vi "Video Displays.vi"() -> ()   [LabVIEW 2017]
uses:
  VideoWindowsCommand.ctl
panel:
  in  "Video Feed 2":enum16{"Camera 1", "Camera2", "Mobile"}(ring)=enum."Camera2"
  in  "MozillaBrowser 2":refnum<k7>(container)
  in  "Video Feed":enum16{"Camera 1", "Camera2", "Mobile"}(ring)
  in  "MozillaBrowser":refnum<k7>(container)
  in  "Exit":bool
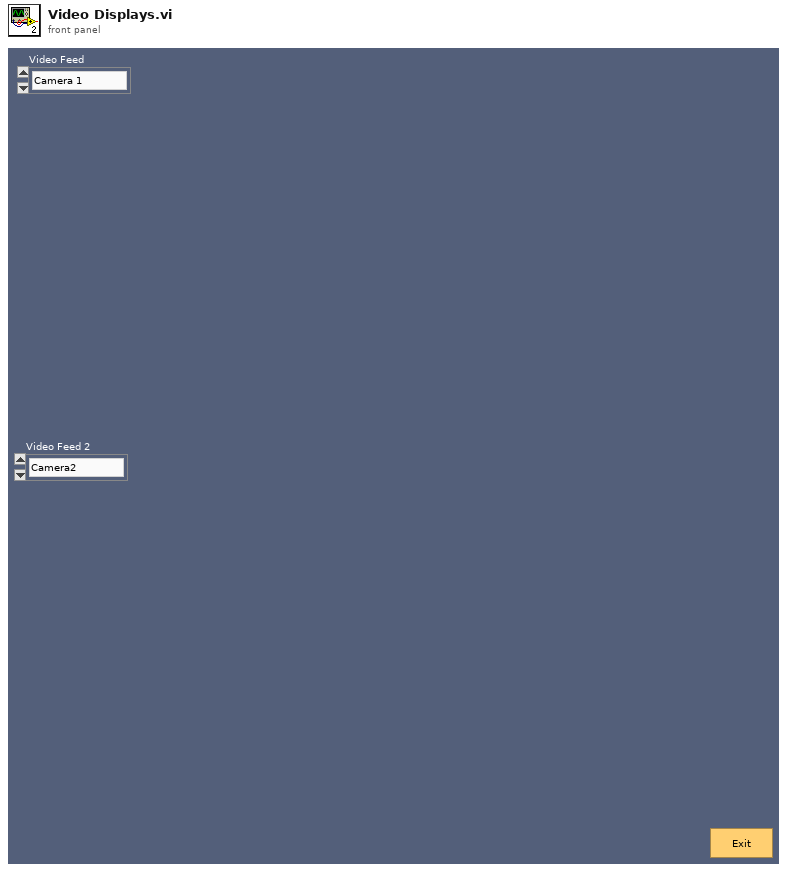
[diagram p1: front panel]
types:
  T1 = typedef "VideoWindowsCommand.ctl" = cluster{"Position":cluster{"Right":i32, "Bottom":i32}, "Exit":bool, "MoveToFront":bool}
  T2 = typedef "LVRectTypeDef.ctl" = cluster{"Left":i16, "Top":i16, "Right":i16, "Bottom":i16}
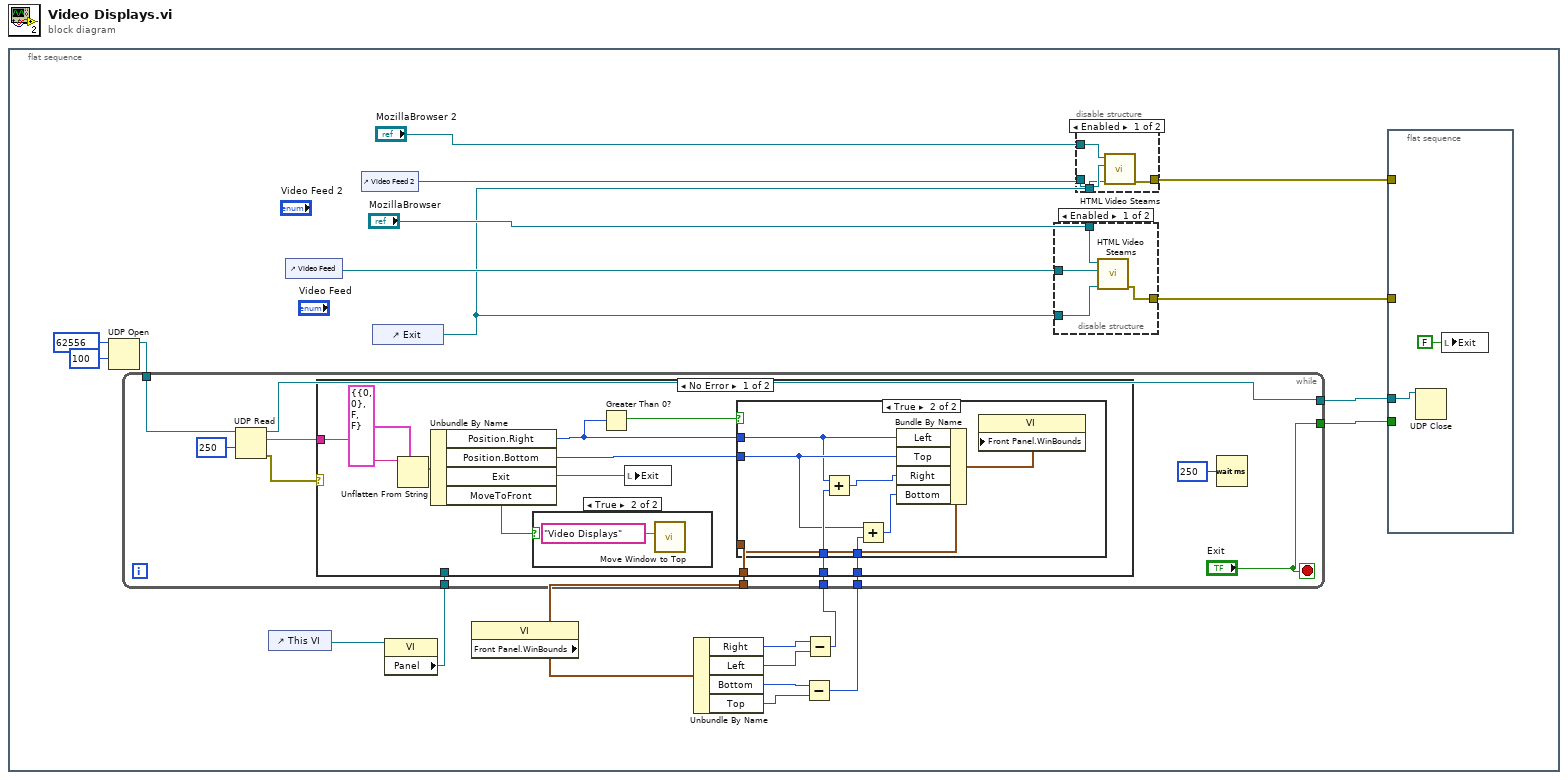
[diagram p0: block diagram]
diagram:
  n1 = flat-sequence {
    frame #0 {
      n2 = UDP Open(9:100 ("timeout ms (25000)"), 11:u16 62556 ("port")) -> (port=w12:refnum<k16>)  [unwired: 3 in, 2 out]
      n3 = control-ref of="This VI"() -> (w11:refnum<vi>)
      n4 = control-ref of="Video Feed"() -> (w20:refnum<vi>)
      n5 = control-ref of="Video Feed 2"() -> (w18:refnum<vi>)
      n6 = control-ref of="Exit"() -> (w14:refnum<vi>)
      n7 = property class="VI"(reference=w11) -> ("Panel"=w10:refnum<vi>)  [unwired: 1 in, 2 out]
      n8 = property class="VI"() -> ("Front Panel.WinBounds"=w3:T2)  [unwired: 2 in, 2 out]
      n9 = Unbundle By Name(w3) -> ("Right"=w6:i16, "Left"=w7:i16, "Bottom"=w4:i16, "Top"=w5:i16)
      n10 = Subtract(x=w4, y=w5) -> (x-y=w1:i16)
      n11 = Subtract(x=w6, y=w7) -> (x-y=w2:i16)
      n12 = while {
        tunnel: ["Exit"] -> w15
        tunnel: w12 -> [w32]
        tunnel: w10 -> [w28]
        tunnel: [w27] -> w9
        tunnel: w3 -> [w26]
        tunnel: w2 -> [w25]
        tunnel: w1 -> [w24]
        stop <- "Exit" stop-if-true
        n13 = UDP Read(connection ID=w32, timeout ms (25000)=250) -> (data out=w29:string, error out=w30:errorcluster, 3:w27:refnum<k16>)  [unwired: 2 in, 2 out]
        n14 = case shown="No Error" w30 {
          tunnel: w29 -> [w45 _]
          tunnel: w28 -> [_ _]
          tunnel: w26 -> [w41 _]
          tunnel: w25 -> [w40 _]
          tunnel: w24 -> [w38 _]
          frame No Error {
            n15 = Unflatten From String(type=T1 {"Position"={"Right"=0, "Bottom"=0}, "Exit"=FALSE, "MoveToFront"=FALSE}, binary string=w45) -> (value=w43:T1)  [unwired: 3 in, 2 out]
            n16 = Unbundle By Name(w43) -> ("Position.Right"=w37:i32, "Position.Bottom"=w39:i32, "Exit"=w42:bool, "MoveToFront"=w35:bool)
            n17 = case shown="True" w35 {
              frame False {
              }
              frame True {
                n18 = call "Move Window to Top.vi"("window name (\"\")"="Video Displays" ("window name (\"\")")) -> ()  [unwired: 5 in, 2 out]
              }
            }
            n19 = Greater Than 0?(x=w37) -> (x > 0?=w36:bool)
            n20 = local write "Exit"(w42) -> ()
            n21 = case shown="True" w36 {
              tunnel: w41 -> [_ w54]
              tunnel: w40 -> [_ w53]
              tunnel: w39 -> [_ w51]
              tunnel: w38 -> [_ w50]
              tunnel: w37 -> [_ w47]
              frame False {
              }
              frame True {
                n22 = Add(x=w47, y=w53) -> (x+y=w52:i32)
                n23 = Add(x=w51, y=w50) -> (x+y=w49:i32)
                n24 = Bundle By Name(cluster=w54, "Left"=w47, "Top"=w51, "Right"=w52, "Bottom"=w49) -> (w48:T2)
                n25 = property class="VI"("Front Panel.WinBounds"=w48) -> ()  [unwired: 2 in, 2 out]
              }
            }
          }
          frame Error {
          }
        }
        n26 = Wait (ms)(milliseconds to wait=u32 250) -> ()  [unwired: 1 out]
      }
      n27 = disable-structure shown="Enabled" {
        disable-tunnel: "MozillaBrowser" -> [w58 _]
        disable-tunnel: [w57 _] -> w16
        disable-tunnel: w20 -> [w56 _]
        disable-tunnel: w14 -> [w55 _]
        frame Enabled {
          n28 = call "HTML Video Steams.vi"("Exit"=w55, "Video Feed 2"=w56, "Automation Refnum in"=w58) -> ("error out"=w57:errorcluster)  [unwired: 7 in, 1 out]
        }
        frame Disabled {
        }
      }
      n29 = disable-structure shown="Enabled" {
        disable-tunnel: "MozillaBrowser 2" -> [w62 _]
        disable-tunnel: w18 -> [w61 _]
        disable-tunnel: w14 -> [w60 _]
        disable-tunnel: [w59 _] -> w17
        frame Enabled {
          n30 = call "HTML Video Steams.vi"("Exit"=w60, "Video Feed 2"=w61, "Automation Refnum in"=w62) -> ("error out"=w59:errorcluster)  [unwired: 7 in, 1 out]
        }
        frame Disabled {
        }
      }
      n31 = flat-sequence {
        tunnel: w17 -> [_]
        tunnel: w16 -> [_]
        tunnel: w15 -> [_]
        tunnel: w9 -> [w22]
        frame #0 {
          n32 = UDP Close(connection ID=w22) -> ()  [unwired: 1 in, 2 out]
          n33 = local write "Exit"(FALSE ("Exit")) -> ()
        }
      }
    }
  }
